vi "uTTA_Init.vi"(8 "error in":errorcluster, 10 "MeasurementConfig":T1, 11 "VISA in":refnum<visa-resource-name>) -> (0 "error out":errorcluster, 3 "VISA out":refnum<visa-resource-name>)   [LabVIEW 2021]
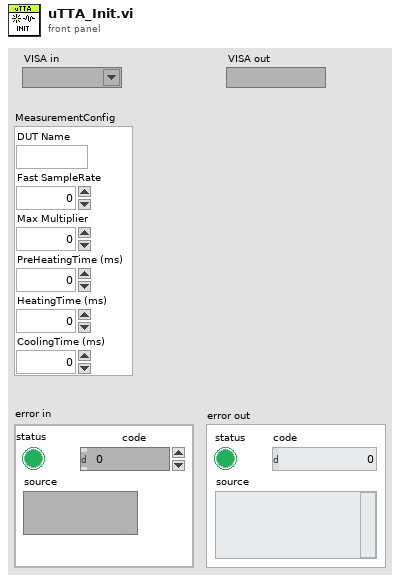
[diagram p1: front panel]
types:
  T1 = cluster{"DUT Name":string, "Fast SampleRate":u16, "Max Multiplier":u16, "PreHeatingTime (ms)":u32, "HeatingTime (ms)":u32, "CoolingTime (ms)":u32}
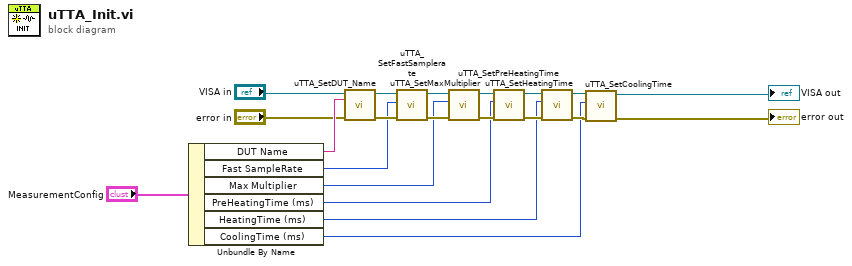
[diagram p0: block diagram]
diagram:
  n1 = Unbundle By Name("MeasurementConfig") -> ("DUT Name"=w20:string, "Fast SampleRate"=w15:u16, "Max Multiplier"=w14:u16, "PreHeatingTime (ms)"=w7:u32, "HeatingTime (ms)"=w6:u32, "CoolingTime (ms)"=w5:u32)
  n2 = call "uTTA_SetDUT_Name.vi"("error in"="error in", "DUT Name"=w20, "VISA Refnum in"="VISA in") -> ("error out"=w18:errorcluster, "VISA Refnum out"=w19:refnum<visa-resource-name>)  [unwired: 6 in, 1 out]
  n3 = call "uTTA_SetFastSamplerate.vi"("error in"=w18, "Fast SampleRate"=w15, "VISA Refnum in"=w19) -> ("error out"=w16:errorcluster, "VISA Refnum out"=w17:refnum<visa-resource-name>)  [unwired: 5 in, 2 out]
  n4 = call "uTTA_SetMaxMultiplier.vi"("error in"=w16, "Max Multiplier"=w14, "VISA Refnum in"=w17) -> ("error out"=w8:errorcluster, "VISA Refnum out"=w13:refnum<visa-resource-name>)  [unwired: 5 in, 2 out]
  n5 = call "uTTA_SetPreHeatingTime.vi"("error in"=w8, "PreHeatingTime (s)"=w7, "VISA Refnum in"=w13) -> ("error out"=w11:errorcluster, "VISA Refnum out"=w12:refnum<visa-resource-name>)  [unwired: 5 in, 2 out]
  n6 = call "uTTA_SetHeatingTime.vi"("error in"=w11, "HeatingTime (s)"=w6, "VISA Refnum in"=w12) -> ("error out"=w9:errorcluster, "VISA Refnum out"=w10:refnum<visa-resource-name>)  [unwired: 5 in, 2 out]
  n7 = call "uTTA_SetCoolingTime.vi"("error in"=w9, "CoolingTime (s)"=w5, "VISA Refnum in"=w10) -> ("error out"=→"error out":errorcluster, "VISA Refnum out"=→"VISA out":refnum<visa-resource-name>)  [unwired: 5 in, 2 out]
